vi "TermostatoDAQ.vi"() -> ()   [LabVIEW 2018]
panel:
  out "Suministro":bool
  out "Temperatura OK":bool
  out "error out 2":errorcluster
  out "error out":errorcluster
  out "Coste del \nsuministro":dbl
  out "Potencia de \nla calefacción":dbl
  out "Consumo":bool
  out "Diferencia de temperatura":dbl[](graph)=[10.459224937438965, 10.476224937438964, 10.460224937438966, 10.477224937438965, 10.462224937438965, 10.482224937438964, 10.459224937438965, 10.456224937438964, 10.472224937438964, 10.458224937438965, 10.474224937438965, 10.459224937438965, 10.473224937438964, 10.459224937438965, 10.474224937438965, 10.461224937438965, 10.484224937438965, 10.460224937438966, 10.457224937438966, 10.472224937438964, 10.458224937438965, 10.474224937438965, 10.461224937438965, 10.476224937438964, 10.459224937438965, 15.556224937438964, 15.559224937438964, 15.557224937438965, 15.558224937438965, 15.559224937438964, 15.558224937438965, 15.559224937438964, 15.558224937438965, 15.559224937438964, 15.558224937438965, 15.559224937438964, 15.557224937438965, 15.559224937438964, 15.559224937438964, 15.558224937438965, 15.559224937438964, 15.558224937438965, 15.559224937438964, 15.558224937438965, 15.559224937438964, 15.557224937438965, 15.559224937438964, 15.559224937438964, 15.558224937438965, 15.559224937438964, 15.558224937438965, 15.559224937438964, 15.558224937438965, 15.559224937438964, 15.557224937438965, 15.559224937438964, 15.559224937438964, 15.558224937438965, 15.559224937438964, 15.557224937438965, 15.559224937438964, 15.558224937438965, 15.559224937438964, 15.558224937438965, 15.559224937438964, 15.558224937438965, 15.558224937438965, 15.559224937438964, 15.558224937438965, 15.559224937438964, 15.558224937438965, 15.559224937438964, 15.558224937438965, 10.457224937438966, 10.475224937438965, 10.459224937438965, 10.459224937438965, 10.471224937438965, 10.457224937438966, 10.473224937438964, 10.459224937438965, 10.474224937438965, 10.461224937438965, 10.476224937438964, 10.460224937438966, 10.469224937438966, 10.467224937438964, 10.459224937438965, 10.475224937438965, 10.460224937438966, 10.474224937438965, 10.460224937438966, 10.477224937438965, 10.462224937438965, 10.482224937438964, 10.462224937438965, 10.458224937438965, 10.474224937438965, 10.458224937438965, 10.475224937438965, 10.461224937438965, 10.475224937438965, 10.460224937438966, 10.474224937438965, 10.461224937438965, 10.484224937438965, 10.459224937438965, 10.459224937438965, 10.475224937438965, 10.458224937438965, 10.475224937438965, 10.460224937438966, 10.475224937438965, 10.460224937438966, 10.476224937438964, 10.459224937438965, 10.473224937438964, 10.461224937438965, 10.459224937438965, 10.476224937438964, 15.559224937438964, 15.557224937438965, 15.559224937438964, 15.557224937438965, 15.559224937438964, 15.557224937438965, 15.559224937438964, 15.559224937438964, 15.558224937438965, 15.559224937438964, 15.558224937438965, 15.559224937438964, 15.558224937438965, 15.559224937438964, 15.557224937438965, 15.559224937438964, 15.559224937438964, 15.558224937438965, 15.559224937438964, 15.558224937438965, 15.559224937438964, 15.558224937438965, 15.559224937438964, 15.558224937438965, 15.559224937438964, 15.558224937438965, 15.559224937438964, 15.559224937438964, 15.558224937438965, 15.559224937438964, 15.558224937438965, 15.559224937438964, 15.558224937438965, 15.559224937438964, 15.557224937438965, 15.559224937438964, 15.559224937438964, 15.558224937438965, 15.559224937438964, 15.558224937438965, 15.559224937438964, 15.558224937438965, 15.559224937438964, 15.557224937438965, 15.559224937438964, 15.559224937438964, 15.558224937438965, 15.559224937438964, 10.467224937438964, 10.458224937438965, 10.472224937438964, 10.460224937438966, 10.474224937438965, 10.461224937438965, 10.468224937438965, 10.464224937438964, 10.458224937438965, 10.473224937438964, 10.460224937438966, 10.477224937438965, 10.460224937438966, 10.477224937438965, 10.461224937438965, 10.481224937438965, 10.461224937438965, 10.459224937438965, 10.475224937438965, 10.458224937438965, 10.476224937438964, 10.460224937438966, 10.477224937438965, 10.462224937438965, 10.479224937438964, 10.462224937438965, 10.484224937438965, 10.459224937438965, 10.459224937438965, 10.473224937438964, 10.459224937438965, 10.475224937438965, 10.458224937438965, 10.474224937438965, 10.459224937438965, 10.476224937438964, 10.461224937438965, 10.472224937438964, 10.463224937438966, 10.459224937438965, 10.473224937438964, 10.459224937438965, 10.474224937438965, 10.461224937438965, 10.475224937438965, 10.460224937438966, 10.479224937438964, 15.559224937438964, 15.559224937438964, 15.557224937438965, 15.559224937438964, 15.557224937438965, 15.559224937438964, 15.558224937438965, 15.559224937438964, 15.558224937438965, 15.559224937438964, 15.558224937438965, 15.558224937438965, 15.559224937438964, 15.558224937438965, 15.559224937438964, 15.558224937438965, 15.559224937438964, 15.558224937438965, 15.559224937438964, 15.557224937438965, 15.559224937438964, 15.559224937438964, 15.558224937438965, 15.559224937438964, 15.558224937438965, 15.559224937438964, 15.558224937438965, 15.559224937438964, 15.557224937438965, 15.559224937438964, 15.559224937438964, 15.558224937438965, 15.559224937438964, 15.558224937438965, 15.559224937438964, 15.558224937438965, 15.559224937438964, 15.558224937438965, 15.559224937438964, 15.559224937438964, 15.558224937438965, 15.559224937438964, 15.558224937438965, 15.559224937438964, 15.558224937438965, 15.559224937438964, 15.557224937438965, 15.559224937438964, 10.467224937438964, 10.465224937438965, 10.458224937438965, 10.471224937438965, 10.458224937438965, 10.473224937438964, 10.460224937438966, 10.476224937438964, 10.459224937438965, 10.480224937438965, 10.461224937438965, 10.459224937438965, 10.474224937438965, 10.461224937438965, 10.475224937438965, 10.459224937438965, 10.476224937438964, 10.461224937438965, 10.476224937438964, 10.463224937438966, 10.486224937438966, 10.459224937438965, 10.458224937438965, 10.473224937438964, 10.459224937438965, 10.475224937438965, 10.461224937438965, 10.476224937438964, 10.460224937438966, 10.478224937438965, 10.461224937438965, 10.469224937438966, 10.468224937438965, 10.459224937438965, 10.473224937438964, 10.458224937438965, 10.474224937438965, 10.461224937438965, 10.479224937438964, 10.462224937438965, 10.481224937438965, 10.460224937438966, 10.456224937438964, 10.473224937438964, 10.459224937438965, 10.475224937438965, 10.458224937438965, 15.557224937438965, 15.559224937438964, 15.557224937438965, 15.559224937438964, 15.557224937438965, 15.559224937438964, 15.559224937438964, 15.558224937438965, 15.559224937438964, 15.558224937438965, 15.559224937438964, 15.558224937438965, 15.559224937438964, 15.557224937438965, 15.559224937438964, 15.559224937438964, 15.558224937438965, 15.559224937438964, 15.558224937438965, 15.559224937438964, 15.558224937438965, 15.559224937438964, 15.557224937438965, 15.559224937438964, 15.559224937438964, 15.558224937438965, 15.559224937438964, 15.558224937438965, 15.559224937438964, 15.558224937438965, 15.559224937438964, 15.558224937438965, 15.559224937438964, 15.558224937438965, 15.558224937438965, 15.559224937438964, 15.558224937438965, 15.559224937438964, 15.558224937438965, 15.559224937438964, 15.558224937438965, 15.559224937438964, 15.557224937438965, 15.559224937438964, 15.559224937438964, 15.558224937438965, 15.559224937438964, 15.558224937438965, 10.457224937438966, 10.469224937438966, 10.460224937438966, 10.478224937438965, 10.458224937438965, 10.455224937438965, 10.472224937438964, 10.459224937438965, 10.475224937438965, 10.461224937438965, 10.473224937438964, 10.459224937438965, 10.475224937438965, 10.461224937438965, 10.486224937438966, 10.460224937438966, 10.458224937438965, 10.474224937438965, 10.459224937438965, 10.475224937438965, 10.460224937438966, 10.477224937438965, 10.461224937438965, 10.476224937438964, 10.461224937438965, 10.466224937438966, 10.472224937438964, 10.459224937438965, 10.475224937438965, 10.459224937438965, 10.475224937438965, 10.461224937438965, 10.476224937438964, 10.461224937438965, 10.482224937438964, 10.460224937438966, 10.456224937438964, 10.473224937438964, 10.458224937438965, 10.474224937438965, 10.460224937438966, 10.475224937438965, 10.461224937438965, 10.475224937438965, 10.461224937438965, 10.485224937438964, 10.461224937438965, 15.559224937438964, 15.557224937438965, 15.559224937438964, 15.557224937438965, 15.559224937438964, 15.557224937438965, 15.559224937438964, 15.557224937438965, 15.559224937438964, 15.559224937438964, 15.558224937438965, 15.559224937438964, 15.558224937438965, 15.559224937438964, 15.558224937438965, 15.559224937438964, 15.558224937438965, 15.559224937438964, 15.558224937438965, 15.558224937438965, 15.559224937438964, 15.558224937438965, 15.559224937438964, 15.558224937438965, 15.559224937438964, 15.558224937438965, 15.559224937438964, 15.557224937438965, 15.559224937438964, 15.559224937438964, 15.558224937438965, 15.559224937438964, 15.558224937438965, 15.559224937438964, 15.558224937438965, 15.559224937438964, 15.557224937438965, 15.559224937438964, 15.559224937438964, 15.558224937438965, 15.559224937438964, 15.557224937438965, 15.559224937438964, 15.558224937438965, 15.559224937438964, 15.557224937438965, 15.559224937438964, 15.559224937438964, 10.465224937438965, 10.456224937438964, 10.470224937438964, 10.459224937438965, 10.473224937438964, 10.459224937438965, 10.474224937438965, 10.460224937438966, 10.485224937438964, 10.459224937438965, 10.458224937438965, 10.473224937438964, 10.458224937438965, 10.474224937438965, 10.459224937438965, 10.477224937438965, 10.462224937438965, 10.478224937438965, 10.461224937438965, 10.466224937438966, 10.471224937438965, 10.459224937438965, 10.476224937438964, 10.461224937438965, 10.474224937438965, 10.460224937438966, 10.476224937438964, 10.460224937438966, 10.482224937438964, 10.461224937438965, 10.458224937438965, 10.473224937438964, 10.458224937438965, 10.474224937438965, 10.459224937438965, 10.475224937438965, 10.460224937438966, 10.474224937438965, 10.461224937438965, 10.485224937438964, 10.459224937438965, 10.458224937438965, 10.474224937438965, 10.458224937438965, 10.473224937438964, 10.459224937438965, 10.476224937438964]
  out "Temperatura\n Deseada":dbl format="%#.1f"
  in  "?":sgl(slide) scale=-5.0..60.0
  in  "?":bool
  out "Temperatura Actual":dbl[](graph)
  # "Termostato Automático con \ncontador de consumo"
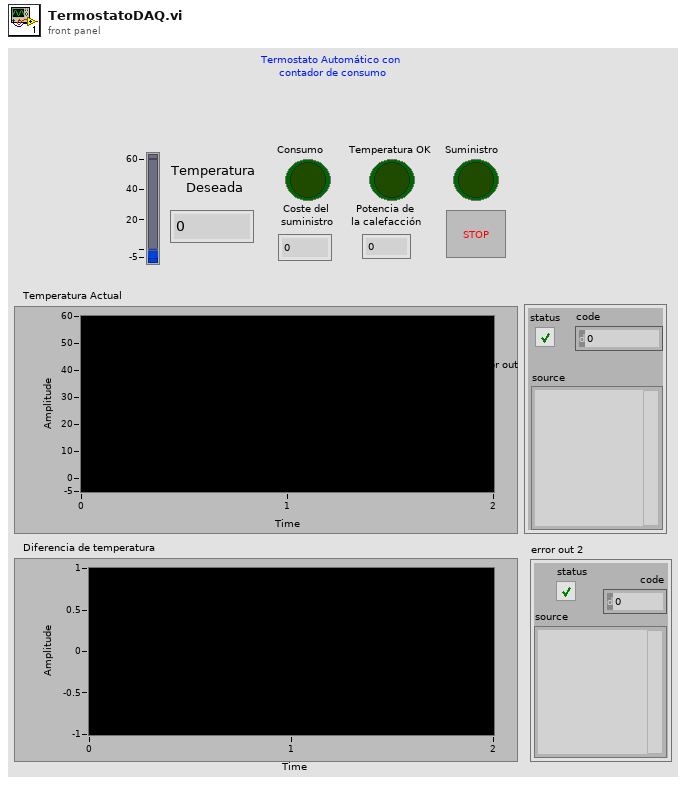
[diagram p1: front panel]
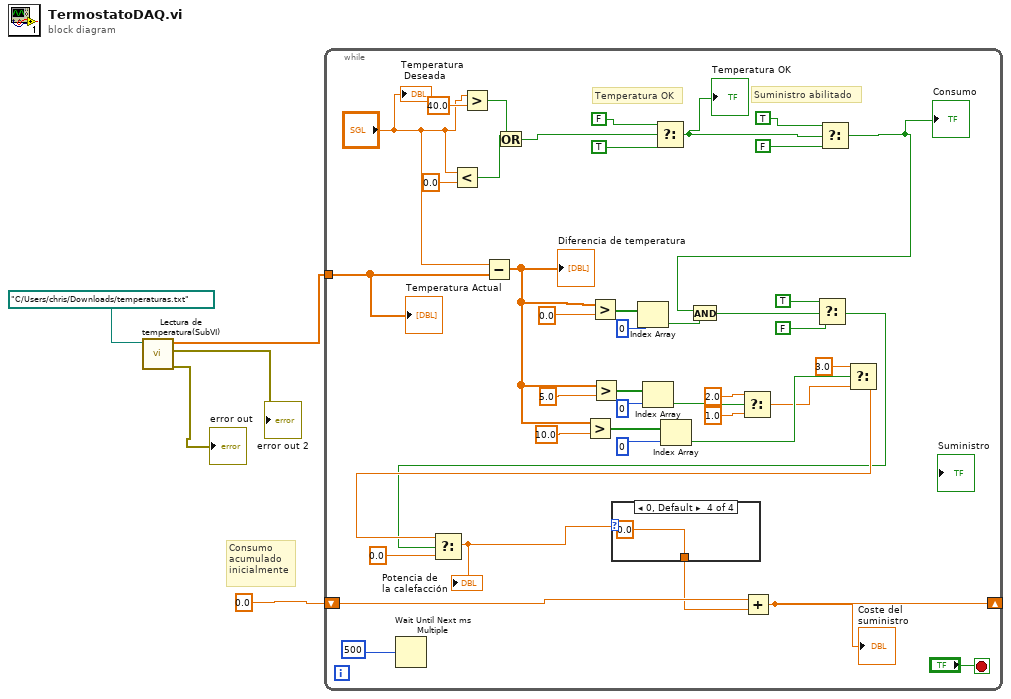
[diagram p0: block diagram]
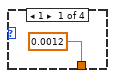
[diagram p2: hidden frame]
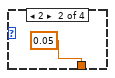
[diagram p3: hidden frame]
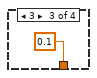
[diagram p4: hidden frame]
diagram:
  # "Consumo\nacumulado\ninicialmente"
  n1 = call "Lectura de temperatura(SubVI).vi"("file path (use dialog)"=path "C:/Users/chris/Downloads/temperaturas.txt") -> ("error out"=→"error out":errorcluster, "error out 2"=→"error out 2":errorcluster, "Array"=w3:dbl[])  [unwired: 8 in]
  n2 = while {
    shift-right: [w11] -> _
    shift-left: 0.0 ("Numeric") -> [w12]
    tunnel: w3 -> [w8]
    stop <- "?" stop-if-true
    # "Suministro abilitado"
    # "Temperatura OK"
    n3 = Wait Until Next ms Multiple(millisecond multiple=u32 500 ("millisecond timer value")) -> ()  [unwired: 1 out]
    n4 = Less?(x="?", y=0.0) -> (x < y?=w38:bool)
    n5 = Greater?(x="?", y=40.0) -> (0:w45:bool)
    n6 = Subtract(x="?", y=w8) -> (x-y=w29:dbl[])
    "Diferencia de temperatura" <- w29
    n7 = Or(x=w38, y=w45) -> (x .or. y?=w46:bool)
    n8 = Greater?(x=w29, y=10.0) -> (0:w24:bool[])
    n9 = Greater?(x=w29, y=0.0) -> (0:w32:bool[])
    n10 = Greater?(x=w29, y=5.0) -> (0:w27:bool[])
    n11 = Index Array(array=w32, index=0) -> (element=w33:bool)
    n12 = Index Array(array=w27, index=0) -> (element=w26:bool)
    n13 = Select(t=FALSE, s=w46, f=TRUE) -> (s? t:f=w7:bool)
    "Temperatura OK" <- w7
    n14 = Index Array(array=w24, index=0) -> (element=w23:bool)
    n15 = Select(t=2.0, s=w26, f=1.0) -> (s? t:f=w19:dbl)
    n16 = Select(t=TRUE, s=w7, f=FALSE) -> (s? t:f=w6:bool)
    "Consumo" <- w6
    n17 = And(x=w6, y=w33) -> (x .and. y?=w9:bool)
    n18 = Select(t=TRUE, s=w9, f=FALSE) -> (s? t:f=w15:bool)
    n19 = Select(t=3.0, s=w23, f=w19) -> (s? t:f=w17:dbl)
    n20 = Select(t=w17, s=w15, f=0.0) -> (s? t:f=w13:dbl)
    "Potencia de \nla calefacción" <- w13
    n21 = case shown="0, Default" w13 {
      tunnel: [0.0012 ("f") 0.05 0.1 ("f") 0.0 ("f")] -> w10
      frame 1 {
      }
      frame 2 {
      }
      frame 3 {
      }
      frame 0, Default {
      }
    }
    n22 = Add(x=w12, y=w10) -> (x+y=w11:dbl)
    "Coste del \nsuministro" <- w11
    "Temperatura Actual" <- w8
    "Temperatura\n Deseada" <- "?"
  }
